vi "Data_Aquisition_cRIO1.vi"() -> ()   [LabVIEW 2016]
uses:
  <vilib>/Platform/TimedLoop/XDataNode/timing_clust.ctl
  <vilib>/Platform/TimedLoop/XDataNode/nitl_modes.ctl
  <vilib>/Platform/TimedLoop/XDataNode/wakeup.ctl
  <vilib>/Utility/file.llb/Write Delimited Spreadsheet (string).vi
  <vilib>/Platform/TimedLoop/XDataNode/loadnilvce.vi
  <vilib>/Utility/file.llb/Write Delimited Spreadsheet (DBL).vi
  <vilib>/Platform/TimedLoop/XDataNode/XDataNode.xnode
  <vilib>/Platform/TimedLoop/XDataNode/XDNodeRunTimeDep.lvlib
panel:
  in  "Mod 8 Labels":string[][](array[string])=[["M3AO0", "M3AO1", "M3AO2", "M3AO3"], ["R1 Air MFC", "R1 N2 MFC", "N/A", "N/A"]]
  out "File Headers":string[][](array[string])=[["Unix Time Code", "M1AI0", "M1AI1", "M1AI2", "M1AI3", "M1AI4", "M1AI5", "M1AI6", "M1AI7", "M2DO0", "M2DO1", "M2DO3  ", "M2DO4", "M2DO4", "M2DO5", "M2DO6", "M2DO7", "M3AO0", "M3AO1", "M3AO2", "M3AO3", "M4DO0", "M4DO1", "M4DO2", "M4DO3", "M4DO4", "M4DO5", "M4DO6", "M4DO7", "M5AI0", "M5AI1", "M5AI2", "M5AI3", "M5AI4", "M5AI5", "M5AI6", "M5AI7", "M6AI0", "M6AI1", "M6AI2", "M6AI3", "M6AI4", "M6AI5", "M6AI6", "M6AI7", "M6AI8", "M6AI9", "M6AI10", "M6AI11", "M6AI12", "M6AI13", "M6A14", "M6AI15", "M7DO0", "M7DO1", "M7DO3  ", "M7DO4", "M7DO4", "M7DO5", "M7DO6", "M7DO7", "M3AO0", "M3AO1", "M3AO2", "M3AO3"], ["Unix Time Code", "R1 pH", "N/A", "R1 N2  ", "R1 ORP", "R1 Air", "R2 DO", "R2 Air", "R2 N2", "R1 Media Pump", "R1 Water Pump", "R1 Eff Pump", "R1 Gas Pump", "R1 Acid Pump", "R1 Base Pump", "R2 Air Valve", "R1 Release Valve", "R1 Air MFC", "R1 N2 MFC", "N/A", "N/A", "R2 Water Pump", "R2 Media Pump", "R2 Eff Pump", "R2 Acid Pump", "R2 Base Pump", "R2 Gas Pump", "R2 Release Valve", "R2 N2 Valve", "R2 pH", "N/A", "N/A", "N/A", "N/A", "N/A", "N/A", "N/A", "R1 DO ", "N/A", "R1 NH4", "N/A", "R1 CA2+", "N/A", "R1 K", "N/A", "R1 Na", "N/A", "R1 Na (2)", "N/A", "R1 NH4+ (2)", "N/A", "R1 ORP", "N/A", "N/A", "N/A", "N/A", "R2 Water Pump 2", "R2 Floc FAir Valve", "R2 Floc Eff Pump", "R2 Floc Return Pump", "N/A", "R1 Air MFC", "R1 N2 MFC", "N/A", "N/A"]]
  in  "Mod 5 Labels":string[][](array[string])=[["M5AI0", "M5AI1", "M5AI2", "M5AI3", "M5AI4", "M5AI5", "M5AI6", "M5AI7"], ["R2 pH", "N/A", "N/A", "N/A", "N/A", "N/A", "N/A", "N/A"]]
  in  "Mod 7 Labels":string[][](array[string])=[["M7DO0", "M7DO1", "M7DO3  ", "M7DO4", "M7DO4", "M7DO5", "M7DO6", "M7DO7"], ["N/A", "N/A", "N/A", "R2 Water Pump 2", "R2 Floc FAir Valve", "R2 Floc Eff Pump", "R2 Floc Return Pump", "N/A"]]
  in  "Mod 6 Labels":string[][](array[string])=[["M6AI0", "M6AI1", "M6AI2", "M6AI3", "M6AI4", "M6AI5", "M6AI6", "M6AI7", "M6AI16", "M6AI7", "M6AI18", "M6AI19", "M6AI20", "M6AI21", "M6AI22", "M6AI23"], ["R1 DO ", "N/A", "R1 NH4+", "N/A", "R1 Ca2+", "N/A", "R1 K+", "N/A", "R1 Na+", "N/A", "R1 Na+ (2)", "N/A", "R1 NH4+ (2)", "N/A", "R1 ORP", "N/A"]]
  in  "Mod 4 Labels":string[][](array[string])=[["M4DO0", "M4DO1", "M4DO2", "M4DO3", "M4DO4", "M4DO5", "M4DO6", "M4DO7"], ["R2 Water Pump", "R2 Media Pump", "R2 Eff Pump", "R2 Acid Pump", "R2 Base Pump", "R2 Gas Pump", "R2 Release Valve", "R2 N2 Valve"]]
  in  "Mod 3 Labels":string[][](array[string])=[["M3AO0", "M3AO1", "M3AO2", "M3AO3"], ["R1 Air MFC", "R1 N2 MFC", "N/A", "N/A"]]
  in  "Mod 2 Labels":string[][](array[string])=[["M2DO0", "M2DO1", "M2DO3  ", "M2DO4", "M2DO4", "M2DO5", "M2DO6", "M2DO7"], ["R1 Media Pump", "R1 Water Pump", "R1 Eff Pump", "R1 Gas Pump", "R1 Acid Pump", "R1 Base Pump", "R2 Air Valve", "R1 Release Valve"]]
  in  "Mod 1 Labels":string[][](array[string])=[["M1AI0", "M1AI1", "M1AI2", "M1AI3", "M1AI4", "M1AI5", "M1AI6", "M1AI7"], ["R1 pH", "N/A", "R1 N2  ", "R1 ORP", "R1 Air", "R2 DO", "R2 Air", "R2 N2"]]
  in  "Buffer Size":i32=100
  out "Saving?":bool=TRUE
  out "new file path (Not A Path if cancelled)":path=path "u:/_11282017_232736.csv"
  in  "File Name:":string
  out "error out":errorcluster={"status"=TRUE, "code"=9, "source"="Open/Create/Replace File in Write Spreadsheet String.vi->Write Delimited Spreadsheet (string).vi->Data_Aquisition_cRIO1.vi<APPEND>\n/u/_11022017_000820.csv"}
  out "iter number":i32=144
  in  "stop":bool
  out "All data":dbl[][](array[numeric])=[[1511882861.6008382, 0.012073636193, -2.1016100000000688e-07, 0.008168856071, -1.7965300000000585e-07, 0.003988651817, 0.005661930065, 0.003985054065, 0.003995193593, 1.0, 1.0, 0.0, 1.0, 0.0, 0.0, 0.0, 0.0, 0.008532159180999999, 0.003999800568, -8.185100000001624e-08, -9.589499999999309e-08, 0.0, 0.0, 0.0, 0.0, 0.0, 1.0, 0.0, 0.0, 0.01249573824, 4.796399999999973e-07, 4.839120000000034e-07, -1.5727999999999792e-07, 1.814320000000124e-07, 5.260980000000164e-07, -1.2229999999999034e-07, 2.1388399999999763e-07, 0.0063802753044, 0.0212250161166, 0.0835895415366, 0.10237329024660001, 0.19010269560780002, 0.231808817001, 0.30033540387900004, 0.34212335546460004, 0.13228594512300001, 0.132676498314, 0.2301027814746, 0.23451913216140002, 0.1383599771316, 0.1676874221472, -0.37530673833420003, -0.3293578454502, 0.0, 0.0, 0.0, 0.0, 0.0, 0.0, 0.0, 0.0, -0.00023295299999999755, -4.289799999999998e-05, -2.4024000000000528e-05, -0.000164249], [1511882861.6107569, 0.012060851993, 4.4552299999999726e-07, 0.008614715751, -1.7965300000000585e-07, 0.004015219898, 0.0057042456770000005, 0.003984725931000001, 0.003996834118000001, 1.0, 1.0, 0.0, 1.0, 0.0, 0.0, 0.0, 0.0, 0.008532159180999999, 0.003999800568, -8.185100000001624e-08, -9.589499999999309e-08, 0.0, 0.0, 0.0, 0.0, 0.0, 1.0, 0.0, 0.0, 0.012532135140000001, 4.796399999999973e-07, 1.5589599999999868e-07, 1.7079200000001346e-07, 1.814320000000124e-07, 1.97924000000006e-07, 2.059040000000086e-07, -4.4258400000000443e-07, 0.0063802753044, 0.0212250161166, 0.0835895415366, 0.10237329024660001, 0.19010269560780002, 0.231808817001, 0.30033540387900004, 0.34212335546460004, 0.13228594512300001, 0.132676498314, 0.2301027814746, 0.23451913216140002, 0.1383599771316, 0.1676874221472, -0.37530673833420003, -0.3293578454502, 0.0, 0.0, 0.0, 0.0, 0.0, 0.0, 0.0, 0.0, -0.00023295299999999755, -4.289799999999998e-05, -2.4024000000000528e-05, -0.000164249], [1511882861.6308308, 0.012236552793, 4.4552299999999726e-07, 0.008546197609, 1.4830499999998672e-07, 0.003990291822, 0.005537935481, 0.003983741529000001, 0.003994537383, 1.0, 1.0, 0.0, 1.0, 0.0, 0.0, 0.0, 0.0, 0.008532159180999999, 0.003999800568, -8.185100000001624e-08, -9.589499999999309e-08, 0.0, 0.0, 0.0, 0.0, 0.0, 1.0, 0.0, 0.0, 0.012732809940000001, -1.7636000000000453e-07, -1.7211999999999252e-07, -1.5727999999999792e-07, 1.814320000000124e-07, -1.3024999999999083e-07, -1.2229999999999034e-07, 5.421179999999987e-07, 0.0063802753044, 0.0212250161166, 0.0835895415366, 0.10237329024660001, 0.19010269560780002, 0.231808817001, 0.30033540387900004, 0.34212335546460004, 0.13228594512300001, 0.132676498314, 0.2301027814746, 0.23451913216140002, 0.1383599771316, 0.1676874221472, -0.37530673833420003, -0.3293578454502, 0.0, 0.0, 0.0, 0.0, 0.0, 0.0, 0.0, 0.0, -0.00023295299999999755, -4.289799999999998e-05, -2.4024000000000528e-05, -0.000164249], [1511882861.7008352, 0.012076914193, 1.1768100000000197e-07, 0.008545214095, -1.7965300000000585e-07, 0.004097220148000001, 0.005672754989, 0.003984725931000001, 0.003995193593, 1.0, 1.0, 0.0, 1.0, 0.0, 0.0, 0.0, 0.0, 0.008532159180999999, 0.003999800568, -8.185100000001624e-08, -9.589499999999309e-08, 0.0, 0.0, 0.0, 0.0, 0.0, 1.0, 0.0, 0.0, 0.012510821640000001, 4.796399999999973e-07, -1.7211999999999252e-07, -1.5727999999999792e-07, -1.4667999999998823e-07, 1.97924000000006e-07, 2.059040000000086e-07, -4.4258400000000443e-07, 0.0063802753044, 0.0212250161166, 0.0835895415366, 0.10237329024660001, 0.19010269560780002, 0.231808817001, 0.30033540387900004, 0.34212335546460004, 0.13228594512300001, 0.132676498314, 0.2301027814746, 0.23451913216140002, 0.1383599771316, 0.1676874221472, -0.37530673833420003, -0.3293578454502, 0.0, 0.0, 0.0, 0.0, 0.0, 0.0, 0.0, 0.0, -0.00023295299999999755, -4.289799999999998e-05, -2.4024000000000528e-05, -0.000164249], [1511882861.790856, 0.012037578193, 1.1768100000000197e-07, 0.008551770855, 1.4830499999998672e-07, 0.004025715930000001, 0.005595996437, 0.003984725931000001, 0.003996506013000001, 1.0, 1.0, 0.0, 1.0, 0.0, 0.0, 0.0, 0.0, 0.008532159180999999, 0.003999800568, -8.185100000001624e-08, -9.589499999999309e-08, 0.0, 0.0, 0.0, 0.0, 0.0, 1.0, 0.0, 0.0, 0.01253803734, 8.076399999999983e-07, 4.839120000000034e-07, -1.5727999999999792e-07, 1.814320000000124e-07, -1.3024999999999083e-07, 2.059040000000086e-07, -1.143500000000034e-07, 0.0063802753044, 0.0212250161166, 0.0835895415366, 0.10237329024660001, 0.19010269560780002, 0.231808817001, 0.30033540387900004, 0.34212335546460004, 0.13228594512300001, 0.132676498314, 0.2301027814746, 0.23451913216140002, 0.1383599771316, 0.1676874221472, -0.37530673833420003, -0.3293578454502, 0.0, 0.0, 0.0, 0.0, 0.0, 0.0, 0.0, 0.0, -0.00023295299999999755, -4.289799999999998e-05, -2.4024000000000528e-05, -0.000164249], [1511882861.8208232, 0.012164436793000001, 4.4552299999999726e-07, 0.008296057215, 1.4830499999998672e-07, 0.003989963821000001, 0.005658977813000001, 0.003984725931000001, 0.003996177908000001, 1.0, 1.0, 0.0, 1.0, 0.0, 0.0, 0.0, 0.0, 0.008532159180999999, 0.003999800568, -8.185100000001624e-08, -9.589499999999309e-08, 0.0, 0.0, 0.0, 0.0, 0.0, 1.0, 0.0, 0.0, 0.01261476594, 1.516399999999964e-07, 1.5589599999999868e-07, 1.7079200000001346e-07, -1.4667999999998823e-07, 1.97924000000006e-07, 2.059040000000086e-07, -1.143500000000034e-07, 0.0063802753044, 0.0212250161166, 0.0835895415366, 0.10237329024660001, 0.19010269560780002, 0.231808817001, 0.30033540387900004, 0.34212335546460004, 0.13228594512300001, 0.132676498314, 0.2301027814746, 0.23451913216140002, 0.1383599771316, 0.1676874221472, -0.37530673833420003, -0.3293578454502, 0.0, 0.0, 0.0, 0.0, 0.0, 0.0, 0.0, 0.0, -0.00023295299999999755, -4.289799999999998e-05, -2.4024000000000528e-05, -0.000164249], [1511882861.880785, 0.012211312193, -2.1016100000000688e-07, 0.008512430295, -1.7965300000000585e-07, 0.00410771618, 0.005557289133000001, 0.003983741529000001, 0.003994865488, 1.0, 1.0, 0.0, 1.0, 0.0, 0.0, 0.0, 0.0, 0.008532159180999999, 0.003999800568, -8.185100000001624e-08, -9.589499999999309e-08, 0.0, 0.0, 0.0, 0.0, 0.0, 1.0, 0.0, 0.0, 0.01270625004, 1.516399999999964e-07, 4.839120000000034e-07, 4.988640000000113e-07, 1.814320000000124e-07, -1.3024999999999083e-07, -1.2229999999999034e-07, 2.1388399999999763e-07, 0.0063802753044, 0.0212250161166, 0.0835895415366, 0.10237329024660001, 0.19010269560780002, 0.231808817001, 0.30033540387900004, 0.34212335546460004, 0.13228594512300001, 0.132676498314, 0.2301027814746, 0.23451913216140002, 0.1383599771316, 0.1676874221472, -0.37530673833420003, -0.3293578454502, 0.0, 0.0, 0.0, 0.0, 0.0, 0.0, 0.0, 0.0, -0.00023295299999999755, -4.289799999999998e-05, -2.4024000000000528e-05, -0.000164249], [1511882861.9207911, 0.012170992793000001, -2.1016100000000688e-07, 0.008379983743, -1.7965300000000585e-07, 0.003998163846, 0.005555320965, 0.0039843977970000005, 0.003995521698000001, 1.0, 1.0, 0.0, 1.0, 0.0, 0.0, 0.0, 0.0, 0.008532159180999999, 0.003999800568, -8.185100000001624e-08, -9.589499999999309e-08, 0.0, 0.0, 0.0, 0.0, 0.0, 1.0, 0.0, 0.0, 0.01270756164, 4.796399999999973e-07, 1.5589599999999868e-07, 1.7079200000001346e-07, 1.814320000000124e-07, 1.97924000000006e-07, 5.341080000000075e-07, 2.1388399999999763e-07, 0.0063802753044, 0.0212250161166, 0.0835895415366, 0.10237329024660001, 0.19010269560780002, 0.231808817001, 0.30033540387900004, 0.34212335546460004, 0.13228594512300001, 0.132676498314, 0.2301027814746, 0.23451913216140002, 0.1383599771316, 0.1676874221472, -0.37530673833420003, -0.3293578454502, 0.0, 0.0, 0.0, 0.0, 0.0, 0.0, 0.0, 0.0, -0.00023295299999999755, -4.289799999999998e-05, -2.4024000000000528e-05, -0.000164249], [1511882861.930883, 0.012242780993, -2.1016100000000688e-07, 0.008234423671, 4.7626299999999283e-07, 0.004027683936, 0.005489387337, 0.0039853821990000005, 0.003994209278, 1.0, 1.0, 0.0, 1.0, 0.0, 0.0, 0.0, 0.0, 0.008532159180999999, 0.003999800568, -8.185100000001624e-08, -9.589499999999309e-08, 0.0, 0.0, 0.0, 0.0, 0.0, 1.0, 0.0, 0.0, 0.012781011240000001, -1.7636000000000453e-07, 1.5589599999999868e-07, -1.5727999999999792e-07, -1.4667999999998823e-07, 1.97924000000006e-07, 5.341080000000075e-07, 2.1388399999999763e-07, 0.0063802753044, 0.0212250161166, 0.0835895415366, 0.10237329024660001, 0.19010269560780002, 0.231808817001, 0.30033540387900004, 0.34212335546460004, 0.13228594512300001, 0.132676498314, 0.2301027814746, 0.23451913216140002, 0.1383599771316, 0.1676874221472, -0.37530673833420003, -0.3293578454502, 0.0, 0.0, 0.0, 0.0, 0.0, 0.0, 0.0, 0.0, -0.00023295299999999755, -4.289799999999998e-05, -2.4024000000000528e-05, -0.000164249], [1511882861.9608269, 0.012022827193000001, 1.1768100000000197e-07, 0.008413751057, 1.4830499999998672e-07, 0.003990291822, 0.0057229432730000005, 0.003983741529000001, 0.003995521698000001, 1.0, 1.0, 0.0, 1.0, 0.0, 0.0, 0.0, 0.0, 0.008532159180999999, 0.003999800568, -8.185100000001624e-08, -9.589499999999309e-08, 0.0, 0.0, 0.0, 0.0, 0.0, 1.0, 0.0, 0.0, 0.01250951004, 8.076399999999983e-07, 1.5589599999999868e-07, -1.5727999999999792e-07, 1.814320000000124e-07, 1.97924000000006e-07, -1.2229999999999034e-07, 2.1388399999999763e-07, 0.0063802753044, 0.0212250161166, 0.0835895415366, 0.10237329024660001, 0.19010269560780002, 0.231808817001, 0.30033540387900004, 0.34212335546460004, 0.13228594512300001, 0.132676498314, 0.2301027814746, 0.23451913216140002, 0.1383599771316, 0.1676874221472, -0.37530673833420003, -0.3293578454502, 0.0, 0.0, 0.0, 0.0, 0.0, 0.0, 0.0, 0.0, -0.00023295299999999755, -4.289799999999998e-05, -2.4024000000000528e-05, -0.000164249], [1511882862.0107741, 0.012116250193, 4.4552299999999726e-07, 0.008587177359, 1.4830499999998672e-07, 0.004064748049, 0.005715726657, 0.003985710333000001, 0.003994537383, 1.0, 1.0, 0.0, 1.0, 0.0, 0.0, 0.0, 0.0, 0.008532159180999999, 0.003999800568, -8.185100000001624e-08, -9.589499999999309e-08, 0.0, 0.0, 0.0, 0.0, 0.0, 1.0, 0.0, 0.0, 0.01249377084, 4.796399999999973e-07, 1.5589599999999868e-07, 4.988640000000113e-07, 1.814320000000124e-07, 1.97924000000006e-07, -1.2229999999999034e-07, -1.143500000000034e-07, 0.0063802753044, 0.0212250161166, 0.0835895415366, 0.10237329024660001, 0.19010269560780002, 0.231808817001, 0.30033540387900004, 0.34212335546460004, 0.13228594512300001, 0.132676498314, 0.2301027814746, 0.23451913216140002, 0.1383599771316, 0.1676874221472, -0.37530673833420003, -0.3293578454502, 0.0, 0.0, 0.0, 0.0, 0.0, 0.0, 0.0, 0.0, -0.00023295299999999755, -4.289799999999998e-05, -2.4024000000000528e-05, -0.000164249], [1511882862.03096, 0.012256876393, 1.1768100000000197e-07, 0.008542591391, -1.7965300000000585e-07, 0.00399619584, 0.005496275925, 0.003983741529000001, 0.003994209278, 1.0, 1.0, 0.0, 1.0, 0.0, 0.0, 0.0, 0.0, 0.008532159180999999, 0.003999800568, -8.185100000001624e-08, -9.589499999999309e-08, 0.0, 0.0, 0.0, 0.0, 0.0, 1.0, 0.0, 0.0, 0.01275904194, -1.7636000000000453e-07, 1.5589599999999868e-07, 1.7079200000001346e-07, -1.4667999999998823e-07, 1.97924000000006e-07, 5.341080000000075e-07, -1.143500000000034e-07, 0.0063802753044, 0.0212250161166, 0.0835895415366, 0.10237329024660001, 0.19010269560780002, 0.231808817001, 0.30033540387900004, 0.34212335546460004, 0.13228594512300001, 0.132676498314, 0.2301027814746, 0.23451913216140002, 0.1383599771316, 0.1676874221472, -0.37530673833420003, -0.3293578454502, 0.0, 0.0, 0.0, 0.0, 0.0, 0.0, 0.0, 0.0, -0.00023295299999999755, -4.289799999999998e-05, -2.4024000000000528e-05, -0.000164249], [1511882862.0608358, 0.012049051193000001, 4.4552299999999726e-07, 0.008705526877, 1.4830499999998672e-07, 0.004072620073, 0.005682267801, 0.003989647941000001, 0.003993553068, 1.0, 1.0, 0.0, 1.0, 0.0, 0.0, 0.0, 0.0, 0.008532159180999999, 0.003999800568, -8.185100000001624e-08, -9.589499999999309e-08, 0.0, 0.0, 0.0, 0.0, 0.0, 1.0, 0.0, 0.0, 0.012527544540000001, 4.796399999999973e-07, 1.5589599999999868e-07, -4.853519999999958e-07, 1.814320000000124e-07, 1.97924000000006e-07, 5.341080000000075e-07, 2.1388399999999763e-07, 0.0063802753044, 0.0212250161166, 0.0835895415366, 0.10237329024660001, 0.19010269560780002, 0.231808817001, 0.30033540387900004, 0.34212335546460004, 0.13228594512300001, 0.132676498314, 0.2301027814746, 0.23451913216140002, 0.1383599771316, 0.1676874221472, -0.37530673833420003, -0.3293578454502, 0.0, 0.0, 0.0, 0.0, 0.0, 0.0, 0.0, 0.0, -0.00023295299999999755, -4.289799999999998e-05, -2.4024000000000528e-05, -0.000164249], [1511882862.08079, 0.012170664993000001, -2.1016100000000688e-07, 0.008177052021000001, 1.4830499999998672e-07, 0.004049004001000001, 0.005635031769, 0.003984069663, 0.003994865488, 1.0, 1.0, 0.0, 1.0, 0.0, 0.0, 0.0, 0.0, 0.008532159180999999, 0.003999800568, -8.185100000001624e-08, -9.589499999999309e-08, 0.0, 0.0, 0.0, 0.0, 0.0, 1.0, 0.0, 0.0, 0.01265116284, 4.796399999999973e-07, 1.5589599999999868e-07, 1.7079200000001346e-07, -1.4667999999998823e-07, 1.97924000000006e-07, 2.059040000000086e-07, 5.421179999999987e-07, 0.0063802753044, 0.0212250161166, 0.0835895415366, 0.10237329024660001, 0.19010269560780002, 0.231808817001, 0.30033540387900004, 0.34212335546460004, 0.13228594512300001, 0.132676498314, 0.2301027814746, 0.23451913216140002, 0.1383599771316, 0.1676874221472, -0.37530673833420003, -0.3293578454502, 0.0, 0.0, 0.0, 0.0, 0.0, 0.0, 0.0, 0.0, -0.00023295299999999755, -4.289799999999998e-05, -2.4024000000000528e-05, -0.000164249], [1511882862.1007462, 0.012204428393, -2.1016100000000688e-07, 0.008587833035, -1.7965300000000585e-07, 0.004099188154, 0.005528422669, 0.003984725931000001, 0.003993553068, 1.0, 1.0, 0.0, 1.0, 0.0, 0.0, 0.0, 0.0, 0.008532159180999999, 0.003999800568, -8.185100000001624e-08, -9.589499999999309e-08, 0.0, 0.0, 0.0, 0.0, 0.0, 1.0, 0.0, 0.0, 0.01270231524, -1.7636000000000453e-07, -1.7211999999999252e-07, 1.7079200000001346e-07, 1.814320000000124e-07, 1.97924000000006e-07, 5.341080000000075e-07, -1.143500000000034e-07, 0.0063802753044, 0.0212250161166, 0.0835895415366, 0.10237329024660001, 0.19010269560780002, 0.231808817001, 0.30033540387900004, 0.34212335546460004, 0.13228594512300001, 0.132676498314, 0.2301027814746, 0.23451913216140002, 0.1383599771316, 0.1676874221472, -0.37530673833420003, -0.3293578454502, 0.0, 0.0, 0.0, 0.0, 0.0, 0.0, 0.0, 0.0, -0.00023295299999999755, -4.289799999999998e-05, -2.4024000000000528e-05, -0.000164249], [1511882862.110684, 0.012126411993, -2.1016100000000688e-07, 0.008378344553000001, -5.07611000000012e-07, 0.003989307819, 0.005583859401000001, 0.003984069663, 0.003993553068, 1.0, 1.0, 0.0, 1.0, 0.0, 0.0, 0.0, 0.0, 0.008532159180999999, 0.003999800568, -8.185100000001624e-08, -9.589499999999309e-08, 0.0, 0.0, 0.0, 0.0, 0.0, 1.0, 0.0, 0.0, 0.01264165374, 4.796399999999973e-07, 4.839120000000034e-07, -1.5727999999999792e-07, 1.814320000000124e-07, -1.3024999999999083e-07, 2.059040000000086e-07, 5.421179999999987e-07, 0.0063802753044, 0.0212250161166, 0.0835895415366, 0.10237329024660001, 0.19010269560780002, 0.231808817001, 0.30033540387900004, 0.34212335546460004, 0.13228594512300001, 0.132676498314, 0.2301027814746, 0.23451913216140002, 0.1383599771316, 0.1676874221472, -0.37530673833420003, -0.3293578454502, 0.0, 0.0, 0.0, 0.0, 0.0, 0.0, 0.0, 0.0, -0.00023295299999999755, -4.289799999999998e-05, -2.4024000000000528e-05, -0.000164249], [1511882862.1307049, 0.012042822993, 1.1768100000000197e-07, 0.008292123159000001, -1.7965300000000585e-07, 0.0039912758250000005, 0.0056871882210000006, 0.0039853821990000005, 0.003994865488, 1.0, 1.0, 0.0, 1.0, 0.0, 0.0, 0.0, 0.0, 0.008532159180999999, 0.003999800568, -8.185100000001624e-08, -9.589499999999309e-08, 0.0, 0.0, 0.0, 0.0, 0.0, 1.0, 0.0, 0.0, 0.01254361164, 4.796399999999973e-07, 1.5589599999999868e-07, 1.7079200000001346e-07, 1.814320000000124e-07, 1.97924000000006e-07, -1.2229999999999034e-07, -1.143500000000034e-07, 0.0063802753044, 0.0212250161166, 0.0835895415366, 0.10237329024660001, 0.19010269560780002, 0.231808817001, 0.30033540387900004, 0.34212335546460004, 0.13228594512300001, 0.132676498314, 0.2301027814746, 0.23451913216140002, 0.1383599771316, 0.1676874221472, -0.37530673833420003, -0.3293578454502, 0.0, 0.0, 0.0, 0.0, 0.0, 0.0, 0.0, 0.0, -0.00023295299999999755, -4.289799999999998e-05, -2.4024000000000528e-05, -0.000164249], [1511882862.1607718, 0.012190660793000001, -2.1016100000000688e-07, 0.008413751057, -5.07611000000012e-07, 0.003990291822, 0.005591404045000001, 0.0039843977970000005, 0.003995849803000001, 1.0, 1.0, 0.0, 1.0, 0.0, 0.0, 0.0, 0.0, 0.008532159180999999, 0.003999800568, -8.185100000001624e-08, -9.589499999999309e-08, 0.0, 0.0, 0.0, 0.0, 0.0, 1.0, 0.0, 0.0, 0.01261870074, 4.796399999999973e-07, 1.5589599999999868e-07, 1.7079200000001346e-07, 1.814320000000124e-07, -1.3024999999999083e-07, -1.2229999999999034e-07, -1.143500000000034e-07, 0.0063802753044, 0.0212250161166, 0.0835895415366, 0.10237329024660001, 0.19010269560780002, 0.231808817001, 0.30033540387900004, 0.34212335546460004, 0.13228594512300001, 0.132676498314, 0.2301027814746, 0.23451913216140002, 0.1383599771316, 0.1676874221472, -0.37530673833420003, -0.3293578454502, 0.0, 0.0, 0.0, 0.0, 0.0, 0.0, 0.0, 0.0, -0.00023295299999999755, -4.289799999999998e-05, -2.4024000000000528e-05, -0.000164249], [1511882862.190835, 0.012161158793, 7.733649999999926e-07, 0.008663891451, 1.4830499999998672e-07, 0.004128708244, 0.005644544581, 0.0039843977970000005, 0.003995193593, 1.0, 1.0, 0.0, 1.0, 0.0, 0.0, 0.0, 0.0, 0.008532159180999999, 0.003999800568, -8.185100000001624e-08, -9.589499999999309e-08, 0.0, 0.0, 0.0, 0.0, 0.0, 1.0, 0.0, 0.0, 0.01261017534, 4.796399999999973e-07, 1.5589599999999868e-07, 4.988640000000113e-07, 1.814320000000124e-07, -1.3024999999999083e-07, 5.341080000000075e-07, -1.143500000000034e-07, 0.0063802753044, 0.0212250161166, 0.0835895415366, 0.10237329024660001, 0.19010269560780002, 0.231808817001, 0.30033540387900004, 0.34212335546460004, 0.13228594512300001, 0.132676498314, 0.2301027814746, 0.23451913216140002, 0.1383599771316, 0.1676874221472, -0.37530673833420003, -0.3293578454502, 0.0, 0.0, 0.0, 0.0, 0.0, 0.0, 0.0, 0.0, -0.00023295299999999755, -4.289799999999998e-05, -2.4024000000000528e-05, -0.000164249], [1511882862.240684, 0.012211312193, 1.1768100000000197e-07, 0.008276386935, 1.4830499999998672e-07, 0.0040430999830000005, 0.0056478248610000005, 0.003984725931000001, 0.003995193593, 1.0, 1.0, 0.0, 1.0, 0.0, 0.0, 0.0, 0.0, 0.008532159180999999, 0.003999800568, -8.185100000001624e-08, -9.589499999999309e-08, 0.0, 0.0, 0.0, 0.0, 0.0, 1.0, 0.0, 0.0, 0.01259410824, 4.796399999999973e-07, 1.5589599999999868e-07, 1.7079200000001346e-07, -1.4667999999998823e-07, -1.3024999999999083e-07, -1.2229999999999034e-07, 2.1388399999999763e-07, 0.0063802753044, 0.0212250161166, 0.0835895415366, 0.10237329024660001, 0.19010269560780002, 0.231808817001, 0.30033540387900004, 0.34212335546460004, 0.13228594512300001, 0.132676498314, 0.2301027814746, 0.23451913216140002, 0.1383599771316, 0.1676874221472, -0.37530673833420003, -0.3293578454502, 0.0, 0.0, 0.0, 0.0, 0.0, 0.0, 0.0, 0.0, -0.00023295299999999755, -4.289799999999998e-05, -2.4024000000000528e-05, -0.000164249], [1511882862.290882, 0.012266382593, -5.380030000000022e-07, 0.008124597941000001, 4.7626299999999283e-07, 0.0039906198230000006, 0.005491027477, 0.003982757127000001, 0.003993881173, 1.0, 1.0, 0.0, 1.0, 0.0, 0.0, 0.0, 0.0, 0.008532159180999999, 0.003999800568, -8.185100000001624e-08, -9.589499999999309e-08, 0.0, 0.0, 0.0, 0.0, 0.0, 1.0, 0.0, 0.0, 0.01271871024, 4.796399999999973e-07, 8.119280000000082e-07, -1.5727999999999792e-07, 1.814320000000124e-07, 1.97924000000006e-07, 2.059040000000086e-07, 5.421179999999987e-07, 0.0063802753044, 0.0212250161166, 0.0835895415366, 0.10237329024660001, 0.19010269560780002, 0.231808817001, 0.30033540387900004, 0.34212335546460004, 0.13228594512300001, 0.132676498314, 0.2301027814746, 0.23451913216140002, 0.1383599771316, 0.1676874221472, -0.37530673833420003, -0.3293578454502, 0.0, 0.0, 0.0, 0.0, 0.0, 0.0, 0.0, 0.0, -0.00023295299999999755, -4.289799999999998e-05, -2.4024000000000528e-05, -0.000164249], [1511882862.3006902, 0.012189349593, 4.4552299999999726e-07, 0.008577670057000001, 1.4830499999998672e-07, 0.0041109961900000005, 0.005523174221, 0.0039834133950000005, 0.003994537383, 1.0, 1.0, 0.0, 1.0, 0.0, 0.0, 0.0, 0.0, 0.008532159180999999, 0.003999800568, -8.185100000001624e-08, -9.589499999999309e-08, 0.0, 0.0, 0.0, 0.0, 0.0, 1.0, 0.0, 0.0, 0.012717070740000001, 1.516399999999964e-07, 1.5589599999999868e-07, -1.5727999999999792e-07, -1.4667999999998823e-07, 1.97924000000006e-07, 2.059040000000086e-07, 2.1388399999999763e-07, 0.0063802753044, 0.0212250161166, 0.0835895415366, 0.10237329024660001, 0.19010269560780002, 0.231808817001, 0.30033540387900004, 0.34212335546460004, 0.13228594512300001, 0.132676498314, 0.2301027814746, 0.23451913216140002, 0.1383599771316, 0.1676874221472, -0.37530673833420003, -0.3293578454502, 0.0, 0.0, 0.0, 0.0, 0.0, 0.0, 0.0, 0.0, -0.00023295299999999755, -4.289799999999998e-05, -2.4024000000000528e-05, -0.000164249], [1511882862.33079, 0.012065441193000001, 4.4552299999999726e-07, 0.008189182027000001, -1.7965300000000585e-07, 0.004105420173, 0.0055897639050000005, 0.003983741529000001, 0.003994209278, 1.0, 1.0, 0.0, 1.0, 0.0, 0.0, 0.0, 0.0, 0.008532159180999999, 0.003999800568, -8.185100000001624e-08, -9.589499999999309e-08, 0.0, 0.0, 0.0, 0.0, 0.0, 1.0, 0.0, 0.0, 0.012597059340000001, -1.7636000000000453e-07, 4.839120000000034e-07, 1.7079200000001346e-07, -4.7479199999998886e-07, 5.260980000000164e-07, 5.341080000000075e-07, -1.143500000000034e-07, 0.0063802753044, 0.0212250161166, 0.0835895415366, 0.10237329024660001, 0.19010269560780002, 0.231808817001, 0.30033540387900004, 0.34212335546460004, 0.13228594512300001, 0.132676498314, 0.2301027814746, 0.23451913216140002, 0.1383599771316, 0.1676874221472, -0.37530673833420003, -0.3293578454502, 0.0, 0.0, 0.0, 0.0, 0.0, 0.0, 0.0, 0.0, -0.00023295299999999755, -4.289799999999998e-05, -2.4024000000000528e-05, -0.000164249], [1511882862.3607368, 0.012210656593, -2.1016100000000688e-07, 0.008271797203, 4.7626299999999283e-07, 0.0039912758250000005, 0.005594028269, 0.003985054065, 0.003994865488, 1.0, 1.0, 0.0, 1.0, 0.0, 0.0, 0.0, 0.0, 0.008532159180999999, 0.003999800568, -8.185100000001624e-08, -9.589499999999309e-08, 0.0, 0.0, 0.0, 0.0, 0.0, 1.0, 0.0, 0.0, 0.01267083684, 4.796399999999973e-07, 1.5589599999999868e-07, 1.7079200000001346e-07, 1.814320000000124e-07, -1.3024999999999083e-07, 2.059040000000086e-07, -4.4258400000000443e-07, 0.0063802753044, 0.0212250161166, 0.0835895415366, 0.10237329024660001, 0.19010269560780002, 0.231808817001, 0.30033540387900004, 0.34212335546460004, 0.13228594512300001, 0.132676498314, 0.2301027814746, 0.23451913216140002, 0.1383599771316, 0.1676874221472, -0.37530673833420003, -0.3293578454502, 0.0, 0.0, 0.0, 0.0, 0.0, 0.0, 0.0, 0.0, -0.00023295299999999755, -4.289799999999998e-05, -2.4024000000000528e-05, -0.000164249], [1511882862.380828, 0.012231963593, -2.1016100000000688e-07, 0.008249832057, -1.7965300000000585e-07, 0.003989963821000001, 0.005496603953, 0.0039834133950000005, 0.003994537383, 1.0, 1.0, 0.0, 1.0, 0.0, 0.0, 0.0, 0.0, 0.008532159180999999, 0.003999800568, -8.185100000001624e-08, -9.589499999999309e-08, 0.0, 0.0, 0.0, 0.0, 0.0, 1.0, 0.0, 0.0, 0.01279576674, 4.796399999999973e-07, 1.5589599999999868e-07, 1.7079200000001346e-07, 1.814320000000124e-07, -1.3024999999999083e-07, -4.505039999999893e-07, -1.143500000000034e-07, 0.0063802753044, 0.0212250161166, 0.0835895415366, 0.10237329024660001, 0.19010269560780002, 0.231808817001, 0.30033540387900004, 0.34212335546460004, 0.13228594512300001, 0.132676498314, 0.2301027814746, 0.23451913216140002, 0.1383599771316, 0.1676874221472, -0.37530673833420003, -0.3293578454502, 0.0, 0.0, 0.0, 0.0, 0.0, 0.0, 0.0, 0.0, -0.00023295299999999755, -4.289799999999998e-05, -2.4024000000000528e-05, -0.000164249], [1511882862.3908901, 0.012199511393, 1.1768100000000197e-07, 0.008680283351, 1.4830499999998672e-07, 0.004135924266, 0.005548760405, 0.0039843977970000005, 0.003993224963, 1.0, 1.0, 0.0, 1.0, 0.0, 0.0, 0.0, 0.0, 0.008532159180999999, 0.003999800568, -8.185100000001624e-08, -9.589499999999309e-08, 0.0, 0.0, 0.0, 0.0, 0.0, 1.0, 0.0, 0.0, 0.01270428264, -1.7636000000000453e-07, 1.5589599999999868e-07, -1.5727999999999792e-07, 5.095439999999995e-07, 5.260980000000164e-07, 2.059040000000086e-07, 5.421179999999987e-07, 0.0063802753044, 0.0212250161166, 0.0835895415366, 0.10237329024660001, 0.19010269560780002, 0.231808817001, 0.30033540387900004, 0.34212335546460004, 0.13228594512300001, 0.132676498314, 0.2301027814746, 0.23451913216140002, 0.1383599771316, 0.1676874221472, -0.37530673833420003, -0.3293578454502, 0.0, 0.0, 0.0, 0.0, 0.0, 0.0, 0.0, 0.0, -0.00023295299999999755, -4.289799999999998e-05, -2.4024000000000528e-05, -0.000164249], [1511882862.400824, 0.012026105193, 4.4552299999999726e-07, 0.008231800967, -1.7965300000000585e-07, 0.00398963582, 0.005690468501, 0.003984725931000001, 0.003995193593, 1.0, 1.0, 0.0, 1.0, 0.0, 0.0, 0.0, 0.0, 0.008532159180999999, 0.003999800568, -8.185100000001624e-08, -9.589499999999309e-08, 0.0, 0.0, 0.0, 0.0, 0.0, 1.0, 0.0, 0.0, 0.01249442664, 4.796399999999973e-07, 4.839120000000034e-07, 4.988640000000113e-07, -1.4667999999998823e-07, -1.3024999999999083e-07, 2.059040000000086e-07, 2.1388399999999763e-07, 0.0063802753044, 0.0212250161166, 0.0835895415366, 0.10237329024660001, 0.19010269560780002, 0.231808817001, 0.30033540387900004, 0.34212335546460004, 0.13228594512300001, 0.132676498314, 0.2301027814746, 0.23451913216140002, 0.1383599771316, 0.1676874221472, -0.37530673833420003, -0.3293578454502, 0.0, 0.0, 0.0, 0.0, 0.0, 0.0, 0.0, 0.0, -0.00023295299999999755, -4.289799999999998e-05, -2.4024000000000528e-05, -0.000164249], [1511882862.4306579, 0.012066424593, -2.1016100000000688e-07, 0.008554065721, -1.7965300000000585e-07, 0.0039906198230000006, 0.005585171513, 0.003983741529000001, 0.003995193593, 1.0, 1.0, 0.0, 1.0, 0.0, 0.0, 0.0, 0.0, 0.008532159180999999, 0.003999800568, -8.185100000001624e-08, -9.589499999999309e-08, 0.0, 0.0, 0.0, 0.0, 0.0, 1.0, 0.0, 0.0, 0.01261214274, 4.796399999999973e-07, 1.5589599999999868e-07, -1.5727999999999792e-07, 1.814320000000124e-07, 1.97924000000006e-07, -1.2229999999999034e-07, 2.1388399999999763e-07, 0.0063802753044, 0.0212250161166, 0.0835895415366, 0.10237329024660001, 0.19010269560780002, 0.231808817001, 0.30033540387900004, 0.34212335546460004, 0.13228594512300001, 0.132676498314, 0.2301027814746, 0.23451913216140002, 0.1383599771316, 0.1676874221472, -0.37530673833420003, -0.3293578454502, 0.0, 0.0, 0.0, 0.0, 0.0, 0.0, 0.0, 0.0, -0.00023295299999999755, -4.289799999999998e-05, -2.4024000000000528e-05, -0.000164249], [1511882862.450838, 0.012158864193, -2.1016100000000688e-07, 0.008338020479000001, 4.7626299999999283e-07, 0.003991603826, 0.0056104296690000005, 0.0039843977970000005, 0.003994865488, 1.0, 1.0, 0.0, 1.0, 0.0, 0.0, 0.0, 0.0, 0.008535347641, 0.003999800568, -8.185100000001624e-08, -9.589499999999309e-08, 0.0, 0.0, 0.0, 0.0, 0.0, 1.0, 0.0, 0.0, 0.01263935844, 4.796399999999973e-07, 1.5589599999999868e-07, -1.5727999999999792e-07, 5.095439999999995e-07, -1.3024999999999083e-07, -1.2229999999999034e-07, 2.1388399999999763e-07, 0.0063802753044, 0.0212250161166, 0.0835895415366, 0.10237329024660001, 0.19010269560780002, 0.231808817001, 0.30033540387900004, 0.34212335546460004, 0.13228594512300001, 0.132676498314, 0.2301027814746, 0.23451913216140002, 0.1383599771316, 0.1676874221472, -0.37530673833420003, -0.3293578454502, 0.0, 0.0, 0.0, 0.0, 0.0, 0.0, 0.0, 0.0, -0.00023295299999999755, -4.289799999999998e-05, -2.4024000000000528e-05, -0.000164249], [1511882862.470727, 0.012152635993, -2.1016100000000688e-07, 0.008131154701000001, 1.4830499999998672e-07, 0.003990291822, 0.005524486333, 0.003985054065, 0.003995193593, 1.0, 1.0, 0.0, 1.0, 0.0, 0.0, 0.0, 0.0, 0.008535347641, 0.003999800568, -8.185100000001624e-08, -9.589499999999309e-08, 0.0, 0.0, 0.0, 0.0, 0.0, 1.0, 0.0, 0.0, 0.01266690204, 1.1356399999999992e-06, 4.839120000000034e-07, 4.988640000000113e-07, 8.376560000000001e-07, -1.3024999999999083e-07, 2.059040000000086e-07, -1.143500000000034e-07, 0.0063802753044, 0.0212250161166, 0.0835895415366, 0.10237329024660001, 0.19010269560780002, 0.231808817001, 0.30033540387900004, 0.34212335546460004, 0.13228594512300001, 0.132676498314, 0.2301027814746, 0.23451913216140002, 0.1383599771316, 0.1676874221472, -0.37530673833420003, -0.3293578454502, 0.0, 0.0, 0.0, 0.0, 0.0, 0.0, 0.0, 0.0, -0.00023295299999999755, -4.289799999999998e-05, -2.4024000000000528e-05, -0.000164249], [1511882862.5407262, 0.012206067393, 1.1768100000000197e-07, 0.008433421337, -1.7965300000000585e-07, 0.0039906198230000006, 0.005598620661000001, 0.003984725931000001, 0.003994537383, 1.0, 1.0, 0.0, 1.0, 0.0, 0.0, 0.0, 0.0, 0.008535347641, 0.003999800568, -8.185100000001624e-08, -9.589499999999309e-08, 0.0, 0.0, 0.0, 0.0, 0.0, 1.0, 0.0, 0.0, 0.01263017724, 4.796399999999973e-07, 1.5589599999999868e-07, 1.7079200000001346e-07, -1.4667999999998823e-07, -1.3024999999999083e-07, 2.059040000000086e-07, -1.143500000000034e-07, 0.0063802753044, 0.0212250161166, 0.0835895415366, 0.10237329024660001, 0.19010269560780002, 0.231808817001, 0.30033540387900004, 0.34212335546460004, 0.13228594512300001, 0.132676498314, 0.2301027814746, 0.23451913216140002, 0.1383599771316, 0.1676874221472, -0.37530673833420003, -0.3293578454502, 0.0, 0.0, 0.0, 0.0, 0.0, 0.0, 0.0, 0.0, -0.00023295299999999755, -4.289799999999998e-05, -2.4024000000000528e-05, -0.000164249], [1511882862.5609498, 0.012119528193, 1.1768100000000197e-07, 0.008097715225, -8.355690000000045e-07, 0.003990291822, 0.0055484323770000005, 0.003985054065, 0.003994537383, 1.0, 1.0, 0.0, 1.0, 0.0, 0.0, 0.0, 0.0, 0.008535347641, 0.003999800568, -8.185100000001624e-08, -9.589499999999309e-08, 0.0, 0.0, 0.0, 0.0, 0.0, 1.0, 0.0, 0.0, 0.01270034784, 4.796399999999973e-07, 4.839120000000034e-07, -1.5727999999999792e-07, -1.4667999999998823e-07, 1.97924000000006e-07, 5.341080000000075e-07, 2.1388399999999763e-07, 0.0063802753044, 0.0212250161166, 0.0835895415366, 0.10237329024660001, 0.19010269560780002, 0.231808817001, 0.30033540387900004, 0.34212335546460004, 0.13228594512300001, 0.132676498314, 0.2301027814746, 0.23451913216140002, 0.1383599771316, 0.1676874221472, -0.37530673833420003, -0.3293578454502, 0.0, 0.0, 0.0, 0.0, 0.0, 0.0, 0.0, 0.0, -0.00023295299999999755, -4.289799999999998e-05, -2.4024000000000528e-05, -0.000164249], [1511882862.5707889, 0.012060851993, 1.1768100000000197e-07, 0.008291139645, -5.07611000000012e-07, 0.004089348124, 0.005603541081, 0.003985054065, 0.003995193593, 1.0, 1.0, 0.0, 1.0, 0.0, 0.0, 0.0, 0.0, 0.008535347641, 0.003999800568, -8.185100000001624e-08, -9.589499999999309e-08, 0.0, 0.0, 0.0, 0.0, 0.0, 1.0, 0.0, 0.0, 0.01257082734, 4.796399999999973e-07, 1.5589599999999868e-07, -1.5727999999999792e-07, 1.814320000000124e-07, 1.97924000000006e-07, -1.2229999999999034e-07, 2.1388399999999763e-07, 0.0063802753044, 0.0212250161166, 0.0835895415366, 0.10237329024660001, 0.19010269560780002, 0.231808817001, 0.30033540387900004, 0.34212335546460004, 0.13228594512300001, 0.132676498314, 0.2301027814746, 0.23451913216140002, 0.1383599771316, 0.1676874221472, -0.37530673833420003, -0.3293578454502, 0.0, 0.0, 0.0, 0.0, 0.0, 0.0, 0.0, 0.0, -0.00023295299999999755, -4.289799999999998e-05, -2.4024000000000528e-05, -0.000164249], [1511882862.620719, 0.012014632193, 4.4552299999999726e-07, 0.008281632343, 1.4830499999998672e-07, 0.003988651817, 0.0056816117450000005, 0.003985054065, 0.003997490328000001, 1.0, 1.0, 0.0, 1.0, 0.0, 0.0, 0.0, 0.0, 0.008535347641, 0.003999800568, -8.185100000001624e-08, -9.589499999999309e-08, 0.0, 0.0, 0.0, 0.0, 0.0, 1.0, 0.0, 0.0, 0.01246885044, 4.796399999999973e-07, 1.5589599999999868e-07, 1.7079200000001346e-07, 1.814320000000124e-07, 1.97924000000006e-07, -4.505039999999893e-07, 2.1388399999999763e-07, 0.0063802753044, 0.0212250161166, 0.0835895415366, 0.10237329024660001, 0.19010269560780002, 0.231808817001, 0.30033540387900004, 0.34212335546460004, 0.13228594512300001, 0.132676498314, 0.2301027814746, 0.23451913216140002, 0.1383599771316, 0.1676874221472, -0.37530673833420003, -0.3293578454502, 0.0, 0.0, 0.0, 0.0, 0.0, 0.0, 0.0, 0.0, -0.00023295299999999755, -4.289799999999998e-05, -2.4024000000000528e-05, -0.000164249], [1511882862.650661, 0.012265399193000001, -2.1016100000000688e-07, 0.008464893785, -1.7965300000000585e-07, 0.003989963821000001, 0.005517269717, 0.0039834133950000005, 0.003994209278, 1.0, 1.0, 0.0, 1.0, 0.0, 0.0, 0.0, 0.0, 0.008535347641, 0.003999800568, -8.185100000001624e-08, -9.589499999999309e-08, 0.0, 0.0, 0.0, 0.0, 0.0, 1.0, 0.0, 0.0, 0.01278592974, -1.7636000000000453e-07, 1.5589599999999868e-07, 1.7079200000001346e-07, 1.814320000000124e-07, -1.3024999999999083e-07, 2.059040000000086e-07, 2.1388399999999763e-07, 0.0063802753044, 0.0212250161166, 0.0835895415366, 0.10237329024660001, 0.19010269560780002, 0.231808817001, 0.30033540387900004, 0.34212335546460004, 0.13228594512300001, 0.132676498314, 0.2301027814746, 0.23451913216140002, 0.1383599771316, 0.1676874221472, -0.37530673833420003, -0.3293578454502, 0.0, 0.0, 0.0, 0.0, 0.0, 0.0, 0.0, 0.0, -0.00023295299999999755, -4.289799999999998e-05, -2.4024000000000528e-05, -0.000164249], [1511882862.670817, 0.012060524193000001, -2.1016100000000688e-07, 0.008272452879, -1.7965300000000585e-07, 0.00398963582, 0.005714742573, 0.003984725931000001, 0.003995193593, 1.0, 1.0, 0.0, 1.0, 0.0, 0.0, 0.0, 0.0, 0.008535347641, 0.003999800568, -8.185100000001624e-08, -9.589499999999309e-08, 0.0, 0.0, 0.0, 0.0, 0.0, 1.0, 0.0, 0.0, 0.01247737584, 4.796399999999973e-07, -5.001359999999973e-07, 1.7079200000001346e-07, 1.814320000000124e-07, 5.260980000000164e-07, 2.059040000000086e-07, 5.421179999999987e-07, 0.0063802753044, 0.0212250161166, 0.0835895415366, 0.10237329024660001, 0.19010269560780002, 0.231808817001, 0.30033540387900004, 0.34212335546460004, 0.13228594512300001, 0.132676498314, 0.2301027814746, 0.23451913216140002, 0.1383599771316, 0.1676874221472, -0.37530673833420003, -0.3293578454502, 0.0, 0.0, 0.0, 0.0, 0.0, 0.0, 0.0, 0.0, -0.00023295299999999755, -4.289799999999998e-05, -2.4024000000000528e-05, -0.000164249], [1511882862.700738, 0.012073308393, 7.733649999999926e-07, 0.008582915465, -1.7965300000000585e-07, 0.004109028184, 0.005692108641, 0.003985054065, 0.003995521698000001, 1.0, 1.0, 0.0, 1.0, 0.0, 0.0, 0.0, 0.0, 0.008535347641, 0.003999800568, -8.185100000001624e-08, -9.589499999999309e-08, 0.0, 0.0, 0.0, 0.0, 0.0, 1.0, 0.0, 0.0, 0.012483933840000001, 8.076399999999983e-07, -1.7211999999999252e-07, -1.5727999999999792e-07, -1.4667999999998823e-07, 5.260980000000164e-07, 2.059040000000086e-07, 5.421179999999987e-07, 0.0063802753044, 0.0212250161166, 0.0835895415366, 0.10237329024660001, 0.19010269560780002, 0.231808817001, 0.30033540387900004, 0.34212335546460004, 0.13228594512300001, 0.132676498314, 0.2301027814746, 0.23451913216140002, 0.1383599771316, 0.1676874221472, -0.37530673833420003, -0.3293578454502, 0.0, 0.0, 0.0, 0.0, 0.0, 0.0, 0.0, 0.0, -0.00023295299999999755, -4.289799999999998e-05, -2.4024000000000528e-05, -0.000164249], [1511882862.730739, 0.012039872793, 1.1768100000000197e-07, 0.008306220193000001, -1.7965300000000585e-07, 0.003990291822, 0.005639296133, 0.003984725931000001, 0.003995193593, 1.0, 1.0, 0.0, 1.0, 0.0, 0.0, 0.0, 0.0, 0.008535347641, 0.003999800568, -8.185100000001624e-08, -9.589499999999309e-08, 0.0, 0.0, 0.0, 0.0, 0.0, 1.0, 0.0, 0.0, 0.01254197214, 4.796399999999973e-07, 1.5589599999999868e-07, -4.853519999999958e-07, 1.814320000000124e-07, -1.3024999999999083e-07, -1.2229999999999034e-07, -1.143500000000034e-07, 0.0063802753044, 0.0212250161166, 0.0835895415366, 0.10237329024660001, 0.19010269560780002, 0.231808817001, 0.30033540387900004, 0.34212335546460004, 0.13228594512300001, 0.132676498314, 0.2301027814746, 0.23451913216140002, 0.1383599771316, 0.1676874221472, -0.37530673833420003, -0.3293578454502, 0.0, 0.0, 0.0, 0.0, 0.0, 0.0, 0.0, 0.0, -0.00023295299999999755, -4.289799999999998e-05, -2.4024000000000528e-05, -0.000164249], [1511882862.7409148, 0.012103138193, -2.1016100000000688e-07, 0.008519642731000001, -1.7965300000000585e-07, 0.003993243831, 0.005690796529000001, 0.003983741529000001, 0.003995849803000001, 1.0, 1.0, 0.0, 1.0, 0.0, 0.0, 0.0, 0.0, 0.008535347641, 0.003999800568, -8.185100000001624e-08, -9.589499999999309e-08, 0.0, 0.0, 0.0, 0.0, 0.0, 1.0, 0.0, 0.0, 0.01252787244, 1.516399999999964e-07, -1.7211999999999252e-07, -1.5727999999999792e-07, 5.095439999999995e-07, 1.97924000000006e-07, -1.2229999999999034e-07, 5.421179999999987e-07, 0.0063802753044, 0.0212250161166, 0.0835895415366, 0.10237329024660001, 0.19010269560780002, 0.231808817001, 0.30033540387900004, 0.34212335546460004, 0.13228594512300001, 0.132676498314, 0.2301027814746, 0.23451913216140002, 0.1383599771316, 0.1676874221472, -0.37530673833420003, -0.3293578454502, 0.0, 0.0, 0.0, 0.0, 0.0, 0.0, 0.0, 0.0, -0.00023295299999999755, -4.289799999999998e-05, -2.4024000000000528e-05, -0.000164249], [1511882862.760653, 0.012261137793, -5.380030000000022e-07, 0.008487514607, -1.7965300000000585e-07, 0.003990947824, 0.0055146454930000005, 0.0039843977970000005, 0.003994209278, 1.0, 1.0, 0.0, 1.0, 0.0, 0.0, 0.0, 0.0, 0.008535347641, 0.003999800568, -8.185100000001624e-08, -9.589499999999309e-08, 0.0, 0.0, 0.0, 0.0, 0.0, 1.0, 0.0, 0.0, 0.012768551040000001, 4.796399999999973e-07, -1.7211999999999252e-07, 4.988640000000113e-07, -1.4667999999998823e-07, 5.260980000000164e-07, 2.059040000000086e-07, 2.1388399999999763e-07, 0.0063802753044, 0.0212250161166, 0.0835895415366, 0.10237329024660001, 0.19010269560780002, 0.231808817001, 0.30033540387900004, 0.34212335546460004, 0.13228594512300001, 0.132676498314, 0.2301027814746, 0.23451913216140002, 0.1383599771316, 0.1676874221472, -0.37530673833420003, -0.3293578454502, 0.0, 0.0, 0.0, 0.0, 0.0, 0.0, 0.0, 0.0, -0.00023295299999999755, -4.289799999999998e-05, -2.4024000000000528e-05, -0.000164249], [1511882862.8407898, 0.012166731393, -2.1016100000000688e-07, 0.008473745411000001, 1.4830499999998672e-07, 0.004021123916, 0.005573362505, 0.0039843977970000005, 0.003996506013000001, 1.0, 1.0, 0.0, 1.0, 0.0, 0.0, 0.0, 0.0, 0.008535347641, 0.003999800568, -8.185100000001624e-08, -9.589499999999309e-08, 0.0, 0.0, 0.0, 0.0, 0.0, 1.0, 0.0, 0.0, 0.01271215224, 1.516399999999964e-07, -1.7211999999999252e-07, 4.988640000000113e-07, 1.814320000000124e-07, -1.3024999999999083e-07, 2.059040000000086e-07, -1.143500000000034e-07, 0.006635684692800001, 0.0241299879468, 0.0835337482236, 0.1128165585888, 0.1900927767966, 0.2252363647296, 0.3002957286342, 0.3385563029868, 0.1322375909184, 0.134480482101, 0.23008170400080002, 0.24752269364460003, 0.1383103830756, 0.1754439325056, -0.3753005390772, -0.32869576480260004, 0.0, 0.0, 0.0, 0.0, 0.0, 0.0, 0.0, 0.0, -0.00023295299999999755, -4.289799999999998e-05, -2.4024000000000528e-05, -0.000164249], [1511882862.8507009, 0.012181810193000001, 4.4552299999999726e-07, 0.008583571141, 1.4830499999998672e-07, 0.003991931827, 0.005601244885, 0.003985054065, 0.003994537383, 1.0, 1.0, 0.0, 1.0, 0.0, 0.0, 0.0, 0.0, 0.008535347641, 0.003999800568, -8.185100000001624e-08, -9.589499999999309e-08, 0.0, 0.0, 0.0, 0.0, 0.0, 1.0, 0.0, 0.0, 0.01270821744, 1.516399999999964e-07, 1.5589599999999868e-07, 4.988640000000113e-07, -4.7479199999998886e-07, 1.97924000000006e-07, -1.2229999999999034e-07, -1.143500000000034e-07, 0.006635684692800001, 0.0241299879468, 0.0835337482236, 0.1128165585888, 0.1900927767966, 0.2252363647296, 0.3002957286342, 0.3385563029868, 0.1322375909184, 0.134480482101, 0.23008170400080002, 0.24752269364460003, 0.1383103830756, 0.1754439325056, -0.3753005390772, -0.32869576480260004, 0.0, 0.0, 0.0, 0.0, 0.0, 0.0, 0.0, 0.0, -0.00023295299999999755, -4.289799999999998e-05, -2.4024000000000528e-05, -0.000164249], [1511882862.880817, 0.012124445193, 4.4552299999999726e-07, 0.008495054881, -1.7965300000000585e-07, 0.004096564146, 0.005699653285, 0.0039843977970000005, 0.003995521698000001, 1.0, 1.0, 0.0, 1.0, 0.0, 0.0, 0.0, 0.0, 0.008535347641, 0.003999800568, -8.185100000001624e-08, -9.589499999999309e-08, 0.0, 0.0, 0.0, 0.0, 0.0, 1.0, 0.0, 0.0, 0.01251475644, 4.796399999999973e-07, 1.5589599999999868e-07, -1.5727999999999792e-07, 1.814320000000124e-07, -1.3024999999999083e-07, 5.341080000000075e-07, 5.421179999999987e-07, 0.006635684692800001, 0.0241299879468, 0.0835337482236, 0.1128165585888, 0.1900927767966, 0.2252363647296, 0.3002957286342, 0.3385563029868, 0.1322375909184, 0.134480482101, 0.23008170400080002, 0.24752269364460003, 0.1383103830756, 0.1754439325056, -0.3753005390772, -0.32869576480260004, 0.0, 0.0, 0.0, 0.0, 0.0, 0.0, 0.0, 0.0, -0.00023295299999999755, -4.289799999999998e-05, -2.4024000000000528e-05, -0.000164249]] format="%#3.4f"
  in  "error in":errorcluster
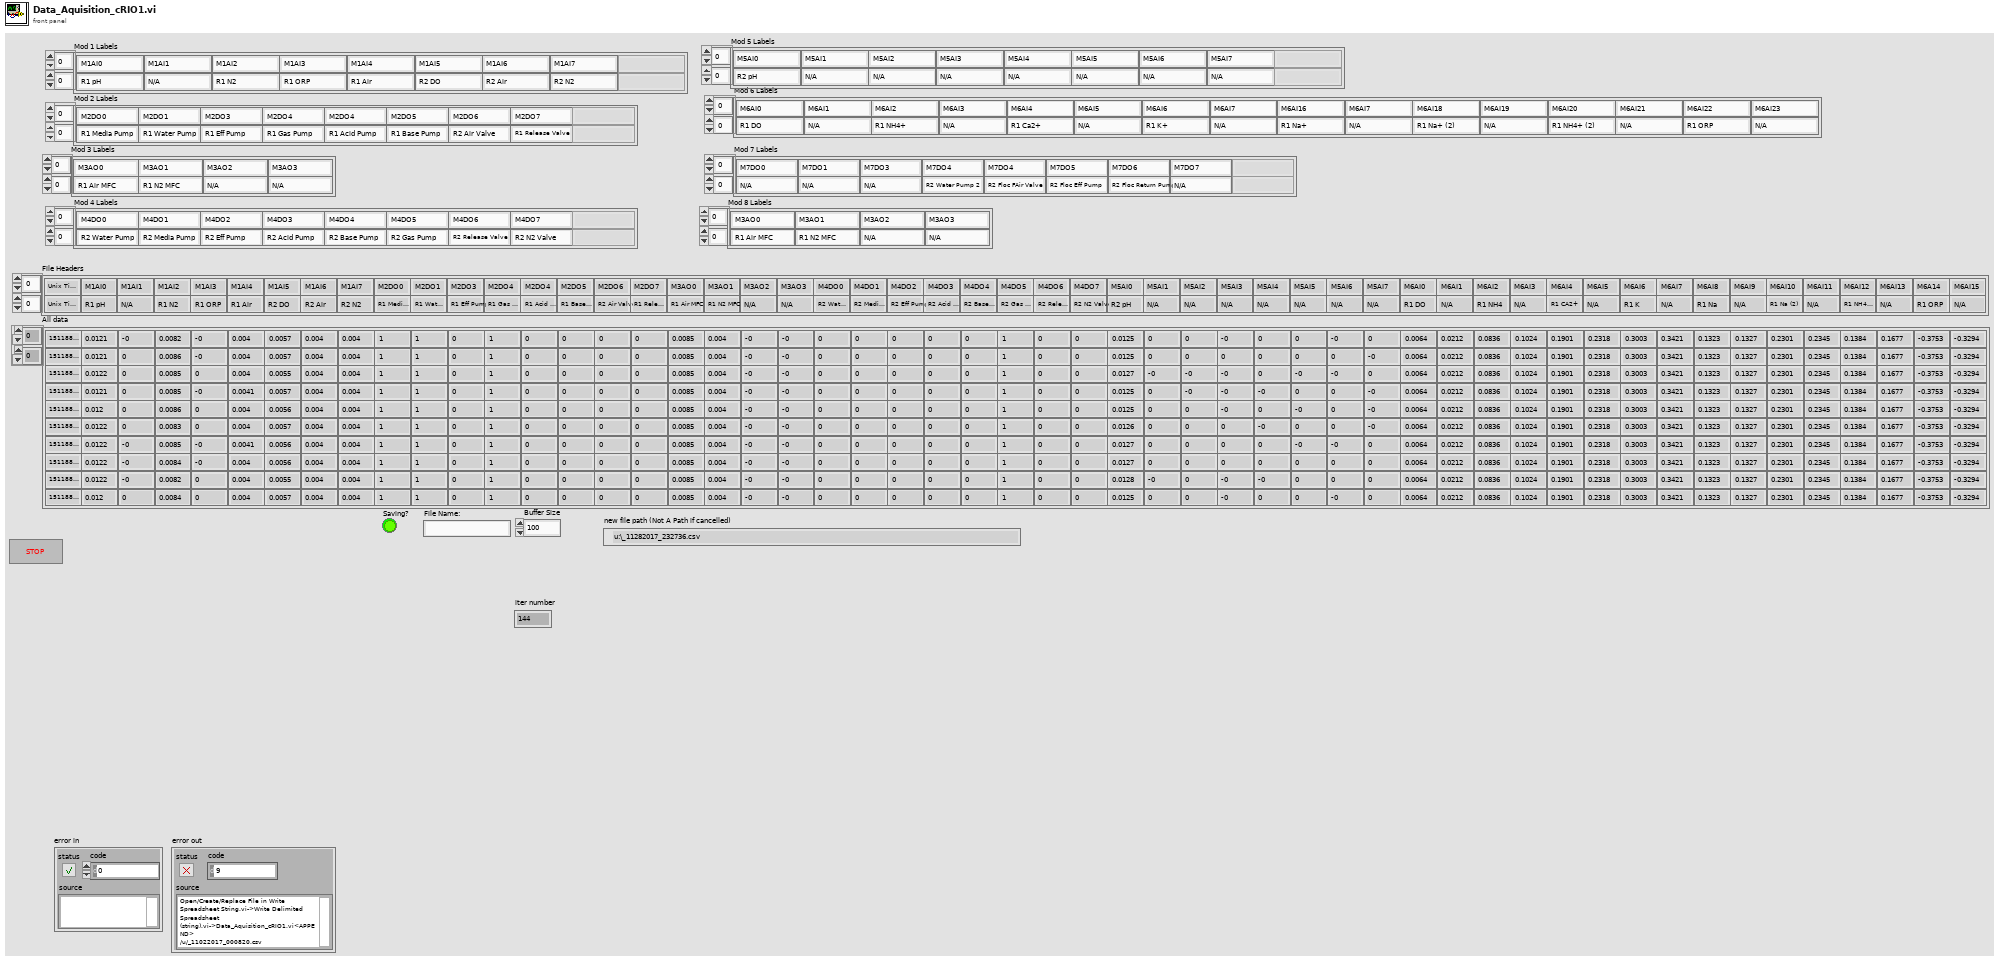
[diagram p1: front panel]
types:
  T1 = typedef "XDNodeRunTimeDep.lvlib/timing_clust.ctl" = cluster{"Expected End [f-1]":u64, "Actual End [f-1]":u64, "Finished Late? [f-1]":bool, "Expected End [i-1]":u64, "Actual End [i-1]":u64, "Finished Late? [i-1]":bool, "Expected Start [i]":u64, "Actual Start [i]":u64, "Expected Start [f]":u64, "Actual Start [f]":u64, "Source Name":string, "Structure Name":string, "Period":i64, "Deadline":i64, "Offset":i64, "Start":i64, "Priority":i32, "Timeout":i32, "Mode":T2, "Wakeup Reason":T3, "Error":errorcluster, "Source Type":string, "Secondary Source Type":string, "Global End Time":u64, "Global Start Time":u64, "Frame Duration":u64, "Iteration Duration":u64, "Assigned CPU":i32, "I/O Scan Engine Mode":u32}
  T2 = typedef "XDNodeRunTimeDep.lvlib/nitl_modes.ctl" = enum32{"No Change", "Process missed periods, maintain original phase", "Discard missed periods, maintain original phase", "Process missed periods, ignore original phase", "Discard missed periods, ignore original phase"}
  T3 = typedef "XDNodeRunTimeDep.lvlib/wakeup.ctl" = enum32{"Normal", "Aborted", "Asynchronous wakeup", "Timing source error", "Timed loop error", "Timeout"}
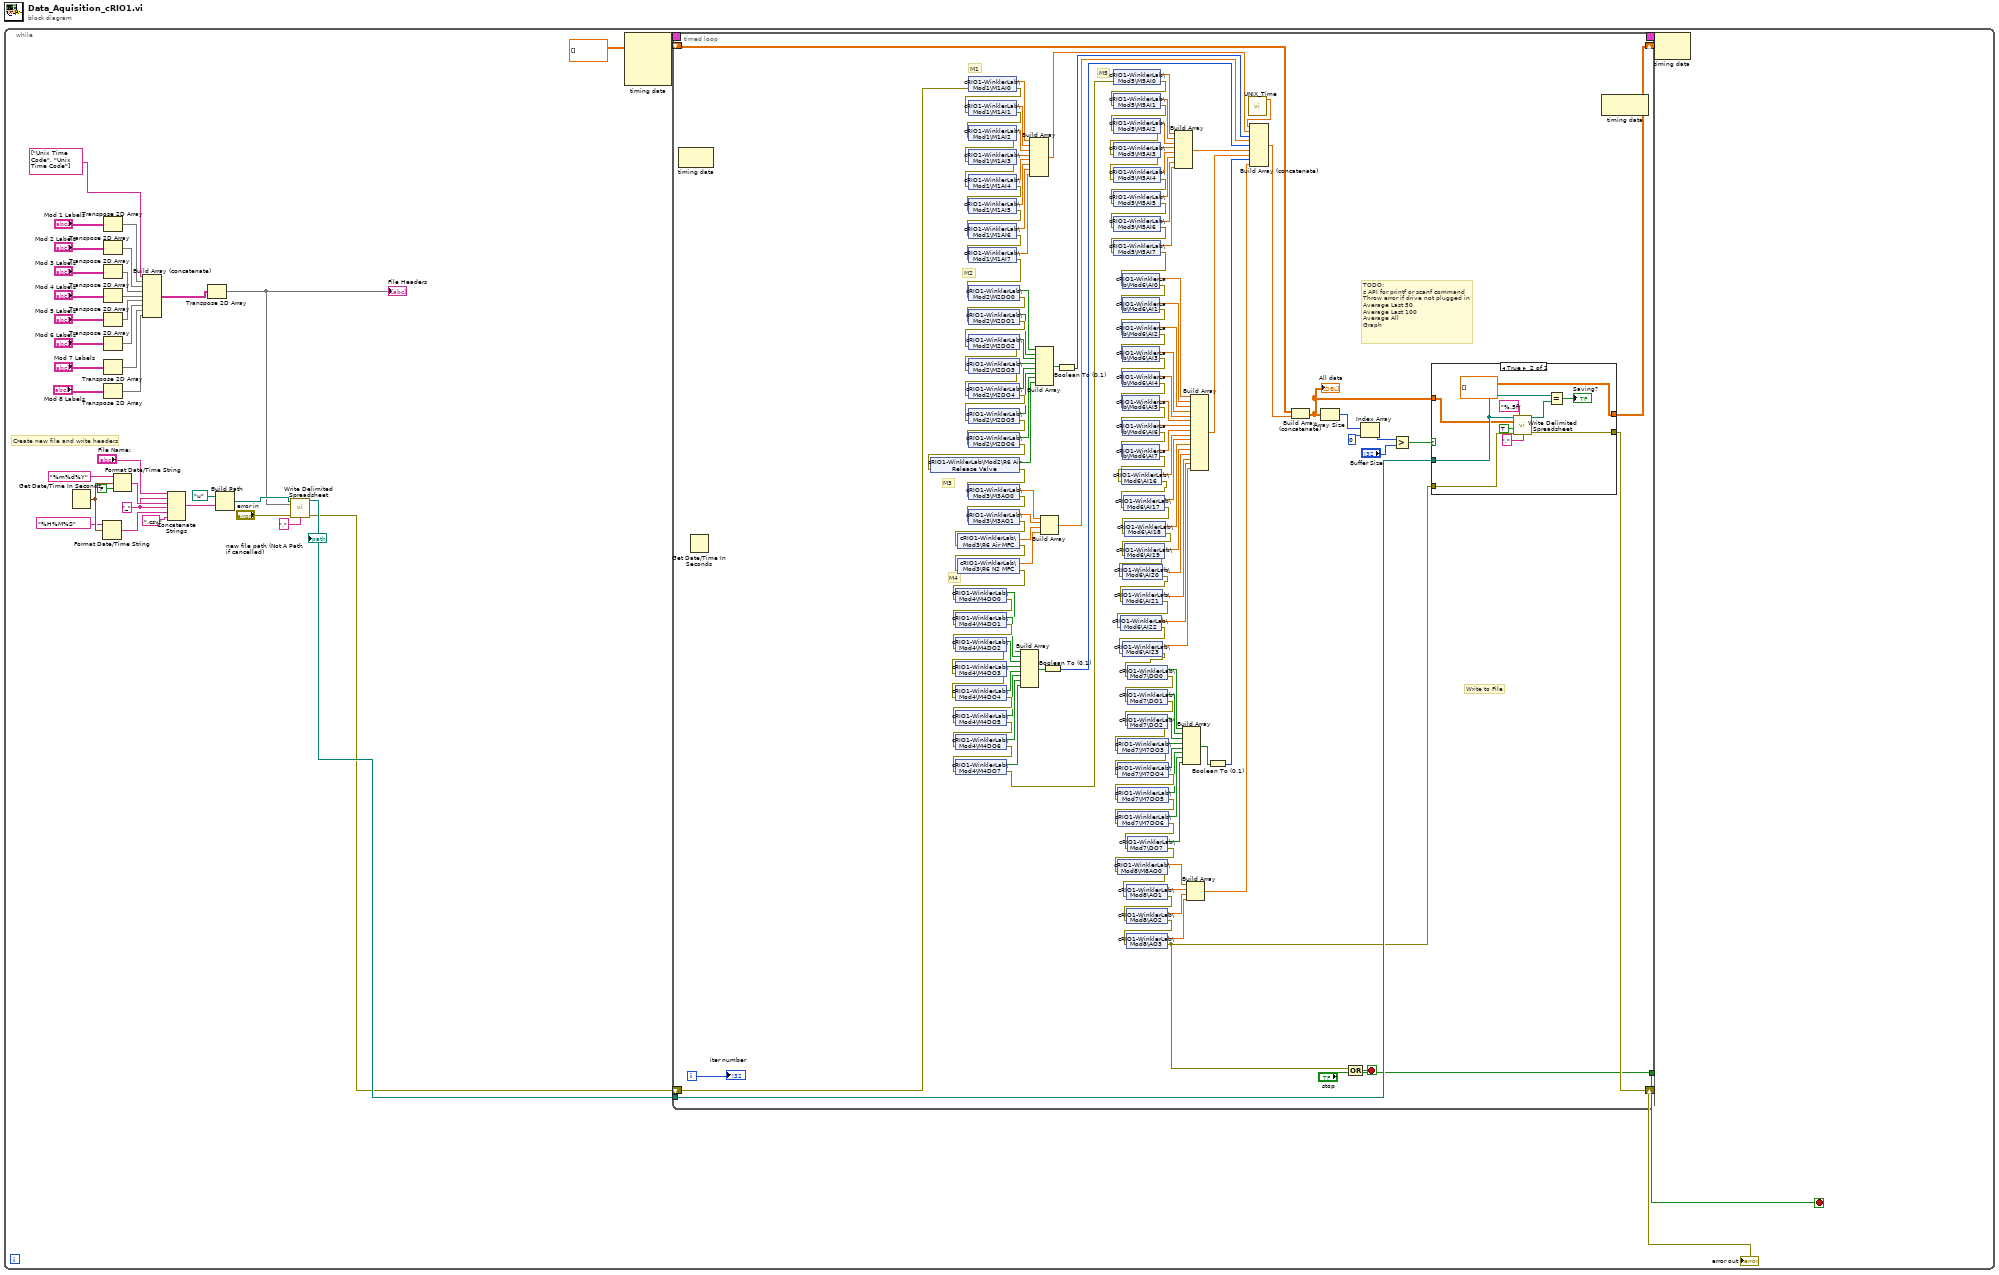
[diagram p0: block diagram]
diagram:
  n1 = while {
    stop <- w25 stop-if-true
    w28 = "_" ("string")
    # "Create new file and write headers"
    n2 = Get Date/Time In Seconds() -> (seconds since 1Jan1904=w33:timestamp)
    n3 = Format Date/Time String(time format string (%c)="%H%M%S", seconds (now)=w33) -> (date/time string=w27:string)  [unwired: 1 in]
    n4 = Transpose 2D Array(2D array="Mod 1 Labels") -> (transposed array=w17:string[][])
    n5 = Transpose 2D Array(2D array="Mod 2 Labels") -> (transposed array=w10:string[][])
    n6 = Transpose 2D Array(2D array="Mod 3 Labels") -> (transposed array=w9:string[][])
    n7 = Transpose 2D Array(2D array="Mod 4 Labels") -> (transposed array=w8:string[][])
    n8 = Transpose 2D Array(2D array="Mod 5 Labels") -> (transposed array=w7:string[][])
    n9 = Transpose 2D Array(2D array="Mod 6 Labels") -> (transposed array=w6:string[][])
    n10 = Transpose 2D Array(2D array="Mod 7 Labels") -> (transposed array=w5:string[][])
    n11 = Transpose 2D Array(2D array="Mod 8 Labels") -> (transposed array=w4:string[][])
    n12 = Format Date/Time String(time format string (%c)="%m%d%Y", seconds (now)=w33, UTC format=FALSE) -> (date/time string=w29:string)
    n13 = Build Array (concatenate)(string[] ["Unix Time Code", "Unix Time Code"], w17, w10, w9, w8, w7, w6, w5, w4) -> (w19:string[][])
    n14 = Concatenate Strings("File Name:", w28, w29, w28, w27, ".csv" ("string")) -> (w26:string)
    n15 = Transpose 2D Array(2D array=w19) -> (transposed array=w2:string[][])
    "File Headers" <- w2
    n16 = Build Path(base path=path "u:/" ("Save to:"), name or relative path=w26) -> (appended path=w36:path)
    n17 = call-poly <vilib>:"Write Delimited Spreadsheet.vi"("file path (dialog if empty)"=w36, "2D data"=w2, "error in (no error)"="error in", "delimiter (\\t)"="," ("delimiter (\\t)")) -> ("new file path (Not A Path if cancelled)"=w40:path, "error out"=w39:errorcluster)  [unwired: 10 in]
    "new file path (Not A Path if cancelled)" <- w40
    n18 = node-c288() -> (w24:T1)  [unwired: 4 in]
    n19 = timed-loop {
      tunnel: w40 -> [w188]
      shift-right: [w64] -> _
      shift-left: dbl[][] [] -> [w193]
      shift-right: [w186] -> w20
      shift-left: w39 -> [w59]
      tunnel: ["stop"] -> w25
      timing: w24 -> [_]
      timing-out: [_] -> w23
      i -> [w194]
      stop <- w195 stop-if-true
      # "M5"
      # "M4"
      # "M3"
      # "M2"
      # "M1"
      # "TODO: \nc API for printf or scanf command\nThrow error if drive not plugged in\nAverage Last 50\nAverage Last 100\nAverage All\nGraph"
      # "Write to File"
      n20 = node-c288() -> ()  [unwired: 1 in, 1 out]
      n21 = Get Date/Time In Seconds() -> ()  [unwired: 1 out]
      n22 = shared-variable "cRIO1-WinklerLab\\Mod1\\M1AI0"(error in=w59) -> (w86:dbl, error out=w92:errorcluster)
      n23 = shared-variable "cRIO1-WinklerLab\\Mod1\\M1AI1"(error in=w92) -> (w87:dbl, error out=w93:errorcluster)
      n24 = shared-variable "cRIO1-WinklerLab\\Mod1\\M1AI2"(error in=w93) -> (w88:dbl, error out=w94:errorcluster)
      n25 = shared-variable "cRIO1-WinklerLab\\Mod1\\M1AI3"(error in=w94) -> (w95:dbl, error out=w96:errorcluster)
      n26 = shared-variable "cRIO1-WinklerLab\\Mod1\\M1AI4"(error in=w96) -> (w89:dbl, error out=w97:errorcluster)
      n27 = shared-variable "cRIO1-WinklerLab\\Mod1\\M1AI5"(error in=w97) -> (w90:dbl, error out=w98:errorcluster)
      n28 = shared-variable "cRIO1-WinklerLab\\Mod1\\M1AI6"(error in=w98) -> (w91:dbl, error out=w99:errorcluster)
      n29 = shared-variable "cRIO1-WinklerLab\\Mod1\\M1AI7"(error in=w99) -> (w61:dbl, error out=w108:errorcluster)
      n30 = shared-variable "cRIO1-WinklerLab\\Mod2\\M2DO0"(error in=w108) -> (w100:bool, error out=w109:errorcluster)
      n31 = shared-variable "cRIO1-WinklerLab\\Mod2\\M2DO1"(error in=w109) -> (w101:bool, error out=w110:errorcluster)
      n32 = shared-variable "cRIO1-WinklerLab\\Mod2\\M2DO2"(error in=w110) -> (w102:bool, error out=w111:errorcluster)
      n33 = shared-variable "cRIO1-WinklerLab\\Mod2\\M2DO3"(error in=w111) -> (w103:bool, error out=w112:errorcluster)
      n34 = shared-variable "cRIO1-WinklerLab\\Mod2\\M2DO4"(error in=w112) -> (w104:bool, error out=w113:errorcluster)
      n35 = shared-variable "cRIO1-WinklerLab\\Mod2\\M2DO5"(error in=w113) -> (w105:bool, error out=w114:errorcluster)
      n36 = shared-variable "cRIO1-WinklerLab\\Mod2\\M2DO6"(error in=w114) -> (w106:bool, error out=w85:errorcluster)
      n37 = shared-variable "cRIO1-WinklerLab\\Mod2\\R6 Air Release Valve"(error in=w85) -> (w107:bool, error out=w120:errorcluster)
      n38 = shared-variable "cRIO1-WinklerLab\\Mod3\\M3AO0"(error in=w120) -> (w115:dbl, error out=w119:errorcluster)
      n39 = shared-variable "cRIO1-WinklerLab\\Mod3\\M3AO1"(error in=w119) -> (w116:dbl, error out=w121:errorcluster)
      n40 = shared-variable "cRIO1-WinklerLab\\Mod3\\R6 Air MFC"(error in=w121) -> (w117:dbl, error out=w122:errorcluster)
      n41 = shared-variable "cRIO1-WinklerLab\\Mod3\\R6 N2 MFC"(error in=w122) -> (w118:dbl, error out=w139:errorcluster)
      n42 = shared-variable "cRIO1-WinklerLab\\Mod4\\M4DO0"(error in=w139) -> (w123:bool, error out=w140:errorcluster)
      n43 = shared-variable "cRIO1-WinklerLab\\Mod4\\M4DO1"(error in=w140) -> (w124:bool, error out=w141:errorcluster)
      n44 = shared-variable "cRIO1-WinklerLab\\Mod4\\M4DO2"(error in=w141) -> (w125:bool, error out=w142:errorcluster)
      n45 = shared-variable "cRIO1-WinklerLab\\Mod4\\M4DO3"(error in=w142) -> (w126:bool, error out=w143:errorcluster)
      n46 = shared-variable "cRIO1-WinklerLab\\Mod4\\M4DO4"(error in=w143) -> (w127:bool, error out=w144:errorcluster)
      n47 = shared-variable "cRIO1-WinklerLab\\Mod4\\M4DO5"(error in=w144) -> (w128:bool, error out=w145:errorcluster)
      n48 = shared-variable "cRIO1-WinklerLab\\Mod4\\M4DO6"(error in=w145) -> (w129:bool, error out=w146:errorcluster)
      n49 = shared-variable "cRIO1-WinklerLab\\Mod4\\M4DO7"(error in=w146) -> (w130:bool, error out=w60:errorcluster)
      n50 = Build Array(w123, w124, w125, w126, w127, w128, w129, w130) -> (w82:bool[])
      n51 = Build Array(w86, w87, w88, w95, w89, w90, w91, w61) -> (w84:dbl[])
      n52 = Build Array(w100, w101, w102, w103, w104, w105, w106, w107) -> (w83:bool[])
      n53 = Build Array(w115, w116, w117, w118) -> (w80:dbl[])
      n54 = Boolean To (0,1)(Boolean=w82) -> (0, 1=w79:i16[])
      n55 = Boolean To (0,1)(Boolean=w83) -> (0, 1=w81:i16[])
      n56 = shared-variable "cRIO1-WinklerLab\\Mod5\\M5AI0"(error in=w60) -> (w131:dbl, error out=w147:errorcluster)
      n57 = shared-variable "cRIO1-WinklerLab\\Mod5\\M5AI1"(error in=w147) -> (w132:dbl, error out=w148:errorcluster)
      n58 = shared-variable "cRIO1-WinklerLab\\Mod5\\M5AI2"(error in=w148) -> (w133:dbl, error out=w149:errorcluster)
      n59 = shared-variable "cRIO1-WinklerLab\\Mod5\\M5AI3"(error in=w149) -> (w134:dbl, error out=w150:errorcluster)
      n60 = shared-variable "cRIO1-WinklerLab\\Mod5\\M5AI4"(error in=w150) -> (w135:dbl, error out=w151:errorcluster)
      n61 = shared-variable "cRIO1-WinklerLab\\Mod5\\M5AI5"(error in=w151) -> (w136:dbl, error out=w152:errorcluster)
      n62 = shared-variable "cRIO1-WinklerLab\\Mod5\\M5AI6"(error in=w152) -> (w137:dbl, error out=w153:errorcluster)
      n63 = shared-variable "cRIO1-WinklerLab\\Mod5\\M5AI7"(error in=w153) -> (w138:dbl, error out=w162:errorcluster)
      n64 = shared-variable "cRIO1-WinklerLab\\Mod6\\AI0"(error in=w162) -> (w154:dbl, error out=w163:errorcluster)
      n65 = shared-variable "cRIO1-WinklerLab\\Mod6\\AI1"(error in=w163) -> (w155:dbl, error out=w164:errorcluster)
      n66 = shared-variable "cRIO1-WinklerLab\\Mod6\\AI2"(error in=w164) -> (w156:dbl, error out=w165:errorcluster)
      n67 = shared-variable "cRIO1-WinklerLab\\Mod6\\AI3"(error in=w165) -> (w157:dbl, error out=w166:errorcluster)
      n68 = shared-variable "cRIO1-WinklerLab\\Mod6\\AI4"(error in=w166) -> (w158:dbl, error out=w167:errorcluster)
      n69 = shared-variable "cRIO1-WinklerLab\\Mod6\\AI5"(error in=w167) -> (w159:dbl, error out=w168:errorcluster)
      n70 = shared-variable "cRIO1-WinklerLab\\Mod6\\AI6"(error in=w168) -> (w160:dbl, error out=w169:errorcluster)
      n71 = shared-variable "cRIO1-WinklerLab\\Mod6\\AI7"(error in=w169) -> (w161:dbl, error out=w50:errorcluster)
      n72 = shared-variable "cRIO1-WinklerLab\\Mod6\\AI16"(error in=w50) -> (w49:dbl, error out=w48:errorcluster)
      n73 = shared-variable "cRIO1-WinklerLab\\Mod6\\AI17"(error in=w48) -> (w51:dbl, error out=w42:errorcluster)
      n74 = shared-variable "cRIO1-WinklerLab\\Mod6\\AI18"(error in=w42) -> (w41:dbl, error out=w43:errorcluster)
      n75 = shared-variable "cRIO1-WinklerLab\\Mod6\\AI19"(error in=w43) -> (w44:dbl, error out=w45:errorcluster)
      n76 = shared-variable "cRIO1-WinklerLab\\Mod6\\AI20"(error in=w45) -> (w47:dbl, error out=w46:errorcluster)
      n77 = shared-variable "cRIO1-WinklerLab\\Mod6\\AI21"(error in=w46) -> (w52:dbl, error out=w53:errorcluster)
      n78 = shared-variable "cRIO1-WinklerLab\\Mod6\\AI22"(error in=w53) -> (w55:dbl, error out=w54:errorcluster)
      n79 = shared-variable "cRIO1-WinklerLab\\Mod6\\AI23"(error in=w54) -> (w57:dbl, error out=w56:errorcluster)
      n80 = shared-variable "cRIO1-WinklerLab\\Mod7\\DO0"(error in=w56) -> (w170:bool, error out=w178:errorcluster)
      n81 = shared-variable "cRIO1-WinklerLab\\Mod7\\DO1"(error in=w178) -> (w171:bool, error out=w179:errorcluster)
      n82 = shared-variable "cRIO1-WinklerLab\\Mod7\\DO2"(error in=w179) -> (w172:bool, error out=w180:errorcluster)
      n83 = shared-variable "cRIO1-WinklerLab\\Mod7\\M7DO3"(error in=w180) -> (w173:bool, error out=w181:errorcluster)
      n84 = shared-variable "cRIO1-WinklerLab\\Mod7\\M7DO4"(error in=w181) -> (w174:bool, error out=w182:errorcluster)
      n85 = shared-variable "cRIO1-WinklerLab\\Mod7\\M7DO5"(error in=w182) -> (w175:bool, error out=w183:errorcluster)
      n86 = shared-variable "cRIO1-WinklerLab\\Mod7\\M7DO6"(error in=w183) -> (w176:bool, error out=w184:errorcluster)
      n87 = shared-variable "cRIO1-WinklerLab\\Mod7\\DO7"(error in=w184) -> (w177:bool, error out=w70:errorcluster)
      n88 = shared-variable "cRIO1-WinklerLab\\Mod8\\M8AO0"(error in=w70) -> (w74:dbl, error out=w69:errorcluster)
      n89 = shared-variable "cRIO1-WinklerLab\\Mod8\\AO1"(error in=w69) -> (w73:dbl, error out=w68:errorcluster)
      n90 = shared-variable "cRIO1-WinklerLab\\Mod8\\AO2"(error in=w68) -> (w72:dbl, error out=w67:errorcluster)
      n91 = shared-variable "cRIO1-WinklerLab\\Mod8\\AO3"(error in=w67) -> (w71:dbl, error out=w62:errorcluster)
      n92 = Build Array(w131, w132, w133, w134, w135, w136, w137, w138) -> (w78:dbl[])
      n93 = Build Array(w170, w171, w172, w173, w174, w175, w176, w177) -> (w76:bool[])
      n94 = Build Array(w74, w73, w72, w71) -> (w66:dbl[])
      n95 = Build Array(w154, w155, w156, w157, w158, w159, w160, w161, w49, w51, w41, w44, w47, w52, w55, w57) -> (w77:dbl[])
      n96 = Boolean To (0,1)(Boolean=w76) -> (0, 1=w75:i16[])
      n97 = call "UNIX_Time.vi"() -> ("Unix time"=w58:dbl)  [unwired: 10 in, 1 out]
      n98 = Build Array (concatenate)(w58, w84, w81, w80, w79, w78, w77, w75, w66) -> (w65:dbl[])
      n99 = Build Array (concatenate)(w193, w65) -> (w63:dbl[][])
      "All data" <- w63
      n100 = Array Size(array=w63) -> (size(s)=w192:i32[])
      n101 = Compound Arithmetic op=OR(w62, "stop") -> (w195:bool)
      n102 = Index Array(array=w192, index=0) -> (element=w190:i32)
      n103 = Greater?(x=w190, y="Buffer Size") -> (0:w189:bool)
      n104 = case shown="True" w189 {
        tunnel: w63 -> [w199 w200]
        tunnel: w188 -> [_ w207]
        tunnel: [w199 dbl[][] []] -> w64
        tunnel: [w198 w206] -> w186
        tunnel: w62 -> [w198 w201]
        frame False {
        }
        frame True {
          n105 = call-poly <vilib>:"Write Delimited Spreadsheet.vi"("file path (dialog if empty)"=w207, "format (%.3f)"="%.5f", "2D data"=w200, "append to file? (new file:F)"=TRUE, "error in (no error)"=w201, "delimiter (\\t)"="," ("delimiter (\\t)")) -> ("new file path (Not A Path if cancelled)"=w208:path, "error out"=w206:errorcluster)  [unwired: 8 in]
          n106 = Equal?(x=w207, y=w208) -> (x = y?=→"Saving?":bool)
        }
      }
      n107 = node-c288() -> ()  [unwired: 1 in, 1 out]
      "iter number" <- w194
    }
    "error out" <- w20
    n108 = node-c288(w23) -> ()  [unwired: 1 out]
  }
